vi "CAN service.vi"(7 "Time Stamp":timestamp format="%<%x %.3X>T", 8 "error in":errorcluster, 9 "Data":u8[](array[numeric]) format="%.0x", 10 "COB-ID":u32 format="%.0x", 11 "CANopen in":refnum<class "CANopen.lvclass">) -> (0 "error out":errorcluster, 3 "CANopen out":refnum<class "CANopen.lvclass">)   [LabVIEW 2024, in "canopen.lvlib" / "CANopen.lvclass"]
doc: "Tries to store the data of a COB (usually an SDO message) into a specific variable. The correct COB-ID must be present inside the provided \"Map\", usually esplicitely requested as a response to an \"SDO upload\". The implementation is quite similar to the PDO handling provided by \"CAN process\", with the notable difference that in this case the entries in the map are consumed."
uses:
  CANopen.lvclass
  CANopen.lvclass/CANopen.ctl
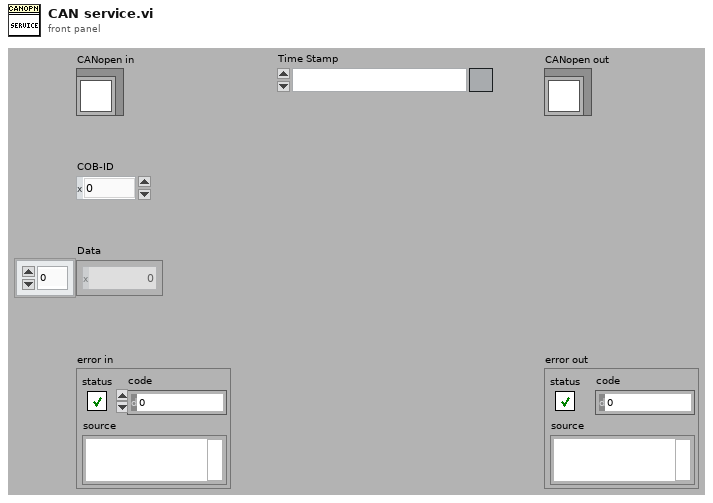
[diagram p1: front panel]
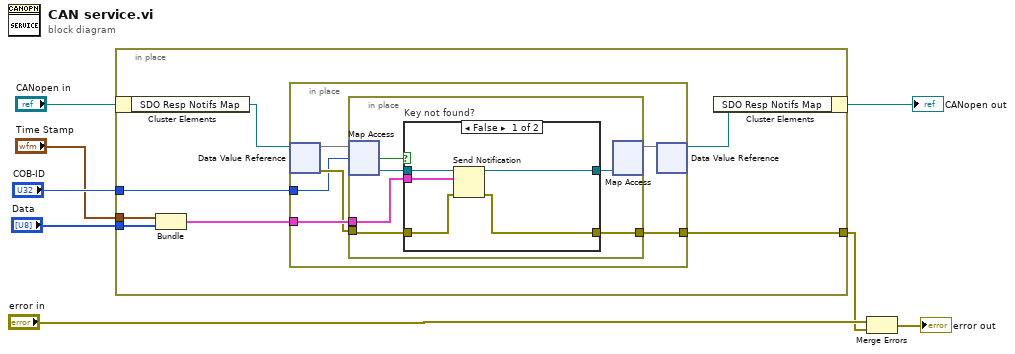
[diagram p0: block diagram]
diagram:
  n1 = in-place {
    in-place-border: "COB-ID" -> [w15]
    in-place-border: "Time Stamp" -> [w14]
    in-place-border: "Data" -> [w13]
    in-place-border: [w9] -> w3
    n2 = in-place-cluster #1("CANopen in") -> ("SDO Resp Notifs Map"=w11:refnum<data-value>)
    n3 = Bundle("Time Stamp"=w14, "Data"=w13) -> (w12:cluster{"Time Stamp":timestamp, "Data":u8[]})  [unwired: 1 in]
    n4 = in-place {
      in-place-border: w15 -> [w16]
      in-place-border: w12 -> [w20]
      in-place-border: [w18] -> w9
      n5 = in-place-dvr #2(w11) -> (w21:map{u32, refnum<notifier>}, w19:errorcluster)
      n6 = in-place {
        in-place-border: w20 -> [w26]
        in-place-border: w19 -> [w24]
        in-place-border: [w23] -> w18
        n7 = in-place-map #3(w21, w16) -> (w27:refnum<notifier>, w25:bool)  [unwired: 1 in]
        n8 = case "Key not found?" shown="False" w25 {
          tunnel: w27 -> [w32 w33]
          tunnel: w26 -> [w31 _]
          tunnel: w24 -> [w30 w34]
          tunnel: [w29 w34] -> w23
          tunnel: [w28 w33] -> w22
          frame False {
            n9 = Send Notification(notification=w31, notifier=w32, error in (no error)=w30) -> (notifier out=w28:refnum<notifier>, error out=w29:errorcluster)
          }
          frame True {
          }
        }
        n10 = in-place-map #3(w22) -> (w17:map{u32, refnum<notifier>})  [unwired: 1 in, 2 out]
      }
      n11 = in-place-dvr #2(w17) -> (w10:refnum<data-value>)  [unwired: 1 out]
    }
    n12 = in-place-cluster #1("SDO Resp Notifs Map"=w10) -> (→"CANopen out":refnum<class "CANopen.lvclass">)
  }
  n13 = Merge Errors("error in", w3) -> (→"error out":errorcluster)
